vi "Main.vi"() -> ()   [LabVIEW 2026]
uses:
  C:/Users/laserfab/Desktop/T-Cube TPZ001-LV2026Q1/Thorlabs.MotionControl.Controls.dll
  Thorlabs.MotionControl.Controls.dll
  <vilib>/numeric/Random Number (Range) DBL.vi
  C:/Users/laserfab/Desktop/T-Cube TPZ001-LV2026Q1/Thorlabs.MotionControl.TCube.PiezoCLI.dll
  Thorlabs.MotionControl.TCube.PiezoCLI.dll
panel:
  out "CloseDevice 2":bool=TRUE
  in  "SerialNumber 2":string="81844656"
  out "GetOutputVoltage 2":dbl=0.00686666463209937
  out "CreateDevice 2":bool=TRUE
  in  "TCubePiezoControl 2":refnum<k24>(container)
  out "GetOutputVoltage":dbl=0.00686666463209937
  out "CloseDevice":bool=TRUE
  in  "stop":bool
  out "CreateDevice":bool=TRUE
  in  "SerialNumber":string="81844665"
  in  "TCubePiezoControl":refnum<k24>(container)
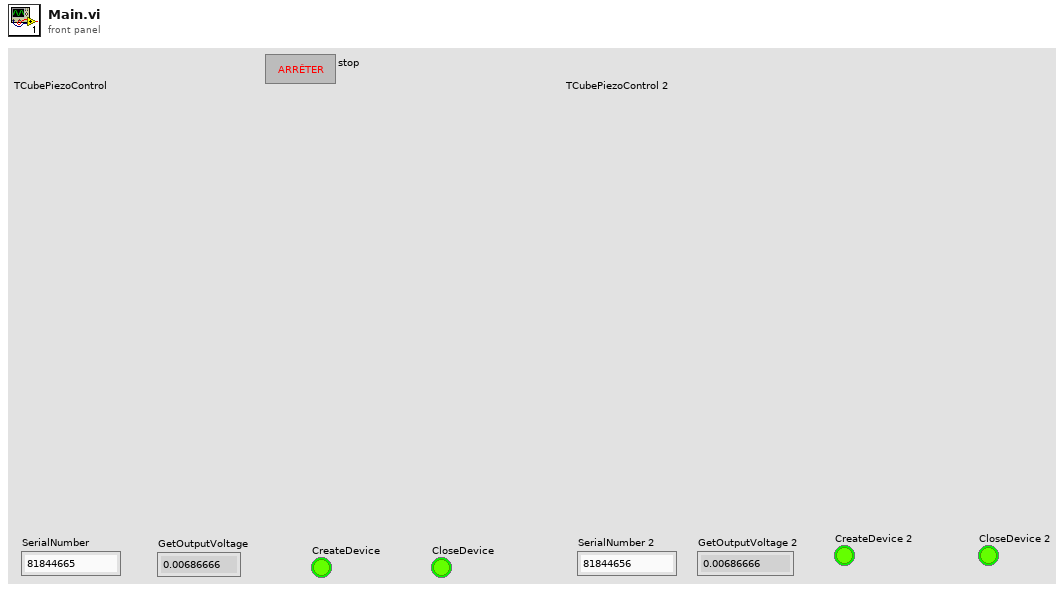
[diagram p1: front panel]
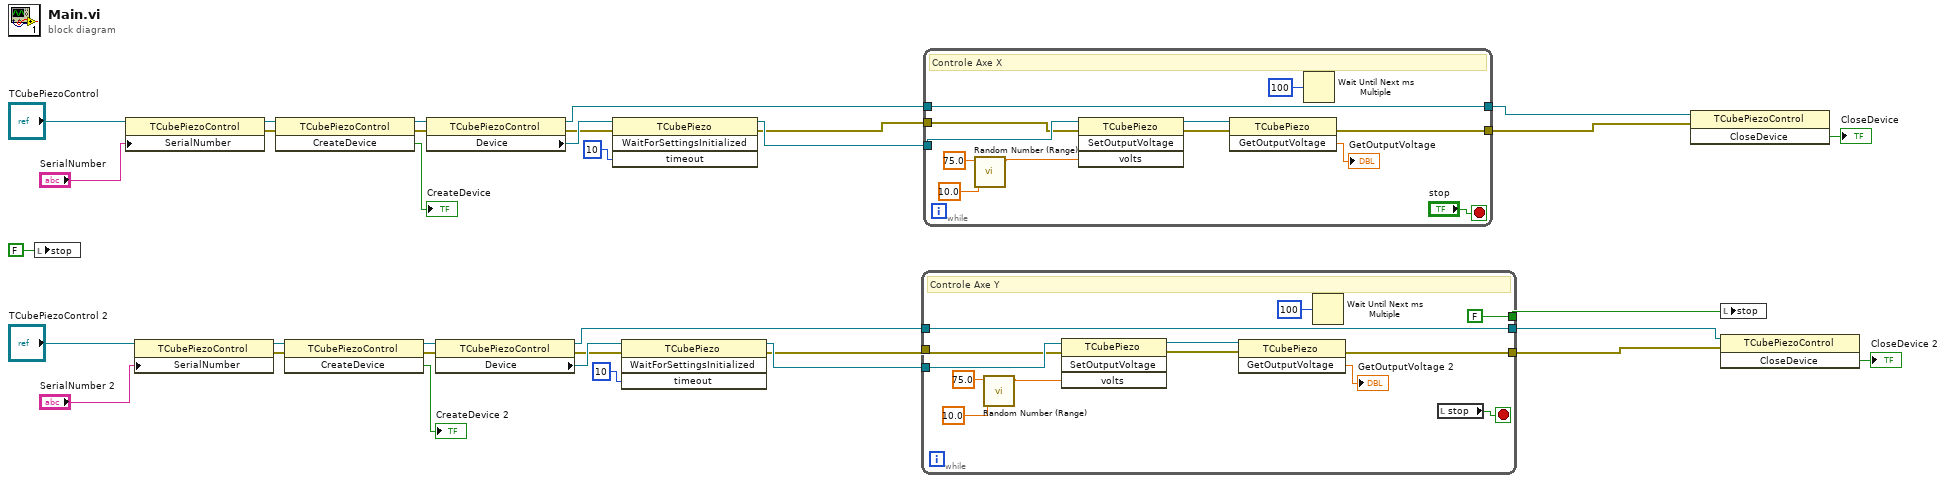
[diagram p0: block diagram]
diagram:
  n1 = local write "stop"(FALSE ("stop")) -> ()
  n2 = property on="Nœud de propriété" class="TCubePiezoControl"(reference="TCubePiezoControl", "SerialNumber"="SerialNumber") -> (reference out=w32:refnum<k24>, error out=w31:errorcluster)  [unwired: 1 in]
  n3 = property on="Nœud de propriété" class="TCubePiezoControl"(reference="TCubePiezoControl 2", "SerialNumber"="SerialNumber 2") -> (reference out=w23:refnum<k24>, error out=w22:errorcluster)  [unwired: 1 in]
  n4 = invoke on="Nœud de méthode" class="TCubePiezoControl" method="CreateDevice"(reference=w32, error in=w31) -> (reference out=w29:refnum<k24>, error out=w30:errorcluster, "CreateDevice"=→"CreateDevice":bool)  [unwired: 1 in]
  n5 = invoke on="Nœud de méthode" class="TCubePiezoControl" method="CreateDevice"(reference=w23, error in=w22) -> (reference out=w20:refnum<k24>, error out=w21:errorcluster, "CreateDevice"=→"CreateDevice 2":bool)  [unwired: 1 in]
  n6 = property on="Nœud de propriété" class="TCubePiezoControl"(reference=w29, error in=w30) -> (reference out=w27:refnum<k24>, error out=w6:errorcluster, "Device"=w7:refnum<k24>)
  n7 = property on="Nœud de propriété" class="TCubePiezoControl"(reference=w20, error in=w21) -> (reference out=w18:refnum<k24>, error out=w8:errorcluster, "Device"=w10:refnum<k24>)
  n8 = invoke on="Nœud de méthode" class="TCubePiezo" method="WaitForSettingsInitialized"(reference=w7, error in=w6, "timeout"=10) -> (reference out=w4:refnum<k24>, error out=w3:errorcluster)  [unwired: 1 in, 2 out]
  n9 = invoke on="Nœud de méthode" class="TCubePiezo" method="WaitForSettingsInitialized"(reference=w10, error in=w8, "timeout"=10) -> (reference out=w2:refnum<k24>, error out=w1:errorcluster)  [unwired: 1 in, 2 out]
  n10 = while {
    tunnel: w18 -> [w47]
    tunnel: [w47] -> w17
    tunnel: [w46] -> w16
    tunnel: [FALSE ("stop")] -> w11
    tunnel: w2 -> [w41]
    tunnel: w1 -> [w40]
    stop <- w43 stop-if-true
    # "Controle Axe Y"
    n11 = call-poly <vilib>:"Random Number (Range).vi"("lower bound (0)"=10.0, "upper bound (100)"=75.0) -> ("number"=w36:dbl)  [unwired: 9 in]
    n12 = invoke on="Nœud de méthode" class="TCubePiezo" method="SetOutputVoltage"(reference=w41, error in=w40, "volts"=w36) -> (reference out=w39:refnum<k24>, error out=w38:errorcluster)  [unwired: 1 in, 2 out]
    n13 = invoke on="Nœud de méthode" class="TCubePiezo" method="GetOutputVoltage"(reference=w39, error in=w38) -> (error out=w46:errorcluster, "GetOutputVoltage"=→"GetOutputVoltage 2":dbl)  [unwired: 1 in, 1 out]
    n14 = Wait Until Next ms Multiple(millisecond multiple=u32 100 ("n millisecondes")) -> ()  [unwired: 1 out]
    n15 = local read "stop"() -> (w43:bool)
  }
  n16 = while {
    tunnel: w27 -> [w59]
    tunnel: [w59] -> w26
    tunnel: [w58] -> w25
    tunnel: w4 -> [w54]
    tunnel: w3 -> [w53]
    stop <- "stop" stop-if-true
    # "Controle Axe X"
    n17 = call-poly <vilib>:"Random Number (Range).vi"("lower bound (0)"=10.0, "upper bound (100)"=75.0) -> ("number"=w49:dbl)  [unwired: 9 in]
    n18 = invoke on="Nœud de méthode" class="TCubePiezo" method="SetOutputVoltage"(reference=w54, error in=w53, "volts"=w49) -> (reference out=w52:refnum<k24>, error out=w51:errorcluster)  [unwired: 1 in, 2 out]
    n19 = invoke on="Nœud de méthode" class="TCubePiezo" method="GetOutputVoltage"(reference=w52, error in=w51) -> (error out=w58:errorcluster, "GetOutputVoltage"=→"GetOutputVoltage":dbl)  [unwired: 1 in, 1 out]
    n20 = Wait Until Next ms Multiple(millisecond multiple=u32 100 ("n millisecondes")) -> ()  [unwired: 1 out]
  }
  n21 = invoke on="Nœud de méthode" class="TCubePiezoControl" method="CloseDevice"(reference=w26, error in=w25) -> ("CloseDevice"=→"CloseDevice":bool)  [unwired: 1 in, 2 out]
  n22 = local write "stop"(w11) -> ()
  n23 = invoke on="Nœud de méthode" class="TCubePiezoControl" method="CloseDevice"(reference=w17, error in=w16) -> ("CloseDevice"=→"CloseDevice 2":bool)  [unwired: 1 in, 2 out]
